vi "Error Status.vi"(8 "error in (no error)":errorcluster, 11 "return value":i32) -> (0 "error out":errorcluster, 3 "return value out":i32)   [LabVIEW 2017, in "libssh2.lvlib"]
uses:
  libssh2.lvlib
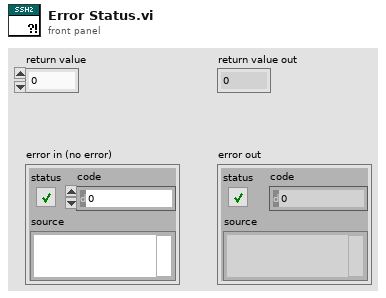
[diagram p1: front panel]
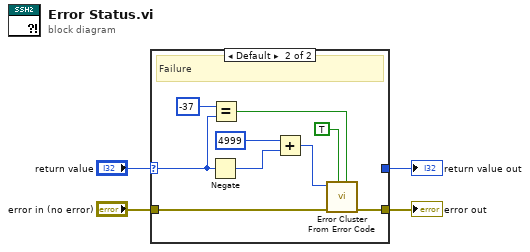
[diagram p0: block diagram]
diagram:
  n1 = case shown="Default" "return value" {
    selector: "return value" -> [w5 w9]
    tunnel: "error in (no error)" -> [w6 w13]
    tunnel: [w6 w12] -> w2
    tunnel: [w5 _] -> w1
    frame 0.. {
      # "Success"
    }
    frame Default {
      # "Failure"
      n2 = Negate(x=w9) -> (-x=w14:i32)
      n3 = Equal?(x=-37, y=w9) -> (x = y?=w7:bool)
      n4 = Add(x=4999 ("return value"), y=w14) -> (x+y=w11:i32)
      n5 = call <vilib>:"Error Cluster From Error Code.vi"("is warning? (False)"=w7, "show call chain? (False)"=TRUE, "error in (no error)"=w13, "error code (0)"=w11) -> ("error out"=w12:errorcluster)  [unwired: 5 in]
    }
  }
  "error out" <- w2
  "return value out" <- w1
